vi "Item Properties.vi"(0 "Tree Reference In":refnum<vi>, 1 "Tag (Current)":string, 5 "error in (no error)":errorcluster, 9 "Column # (0)":i32) -> (14 "Tree Reference Out":refnum<vi>, 15 "Duplicate Tag":string, 16 "Open?":bool, 17 "Child-Only?":bool, 18 "Indent Level":i32, 19 "error out":errorcluster)   [LabVIEW 2010]
doc: "Gets a limited set of properties about the input item"
panel:
  # "VI INPUTS"
  # "VI OUTPUTS"
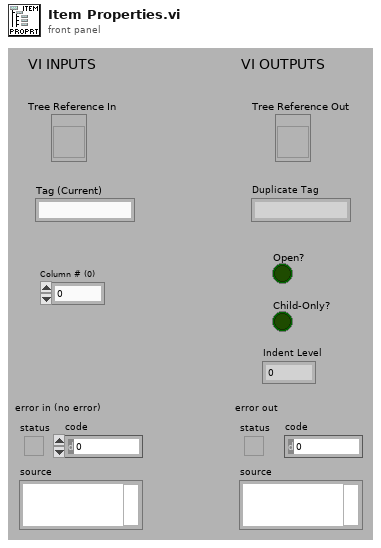
[diagram p1: front panel]
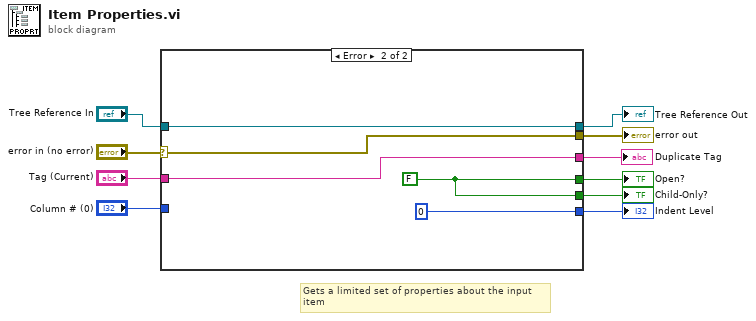
[diagram p0: block diagram]
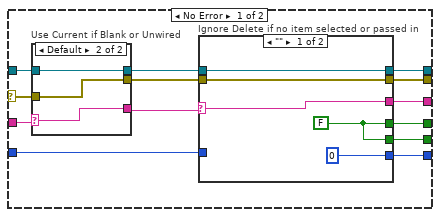
[diagram p2: hidden frame]
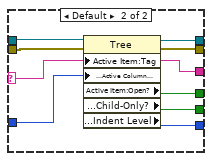
[diagram p3: hidden frame]
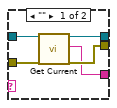
[diagram p4: hidden frame]
diagram:
  # "Gets a limited set of properties about the input item"
  n1 = case shown="Error" "error in (no error)" {
    selector: "error in (no error)" -> [w21 w49]
    tunnel: "Tree Reference In" -> [w23 w50]
    tunnel: [w20 w50] -> w9
    tunnel: [w19 w49] -> w8
    tunnel: "Tag (Current)" -> [w22 w46]
    tunnel: "Column # (0)" -> [w15 _]
    tunnel: [w14 w48] -> w4
    tunnel: [w13 w48] -> w3
    tunnel: [w12 0 ("Indent Level")] -> w2
    tunnel: [w11 w46] -> w1
    frame No Error {
      n2 = case "Use Current if Blank or Unwired" shown="Default" w22 {
        selector: w22 -> [_ w43]
        tunnel: [w41 w45] -> w18
        tunnel: w23 -> [w42 w45]
        tunnel: [w40 w44] -> w17
        tunnel: w21 -> [w39 w44]
        tunnel: [w38 w43] -> w16
        frame "" {
          n3 = call <userlib>:"Get Current.vi"("Tree Reference In"=w42, "error in (no error)"=w39) -> ("Tree Reference Out"=w41:refnum<vi>, "Current Tag"=w38:string, "error out"=w40:errorcluster)  [unwired: 14 in, 1 out]
        }
        frame Default {
        }
      }
      n4 = case "Ignore Delete if no item selected or passed in" shown="\"\"" w16 {
        selector: w16 -> [w24 w29]
        tunnel: [w28 w31] -> w20
        tunnel: [w27 w30] -> w19
        tunnel: w18 -> [w28 w37]
        tunnel: w17 -> [w27 w36]
        tunnel: w15 -> [_ w35]
        tunnel: [w26 w34] -> w14
        tunnel: [w26 w33] -> w13
        tunnel: [0 ("Indent Level") w32] -> w12
        tunnel: [w24 w29] -> w11
        frame "" {
          w26 = FALSE ("Open?")
        }
        frame Default {
          n5 = property class="Tree"(reference=w37, error in=w36, "Active Item:Tag"=w29, "Active Cell:Active Column Number"=w35) -> (reference out=w31:refnum<vi>, error out=w30:errorcluster, "Active Item:Open?"=w34:bool, "Active Item:Child-Only?"=w33:bool, "Active Item:Indent Level"=w32:i32)
        }
      }
    }
    frame Error {
      w48 = FALSE ("Open?")
    }
  }
  "Tree Reference Out" <- w9
  "error out" <- w8
  "Open?" <- w4
  "Child-Only?" <- w3
  "Indent Level" <- w2
  "Duplicate Tag" <- w1
